vi "appendCsvFile.vi"(8 "error in (no error)":errorcluster, 10 "text to write":string, 11 "Byte Stream File in":refnum<file>) -> (0 "error out":errorcluster)   [LabVIEW 2019]
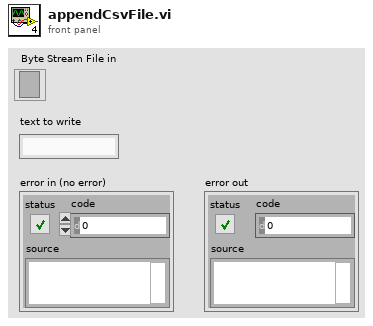
[diagram p1: front panel]
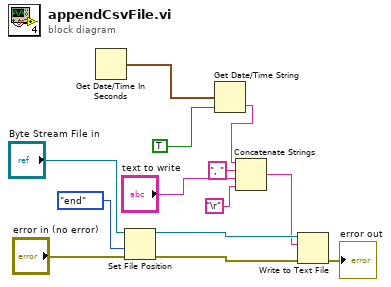
[diagram p0: block diagram]
diagram:
  n1 = Get Date/Time In Seconds() -> (seconds since 1Jan1904=w3:timestamp)
  n2 = Set File Position(refnum="Byte Stream File in", from (0:start)=enum16{"start", "end", "current"}."end", error in="error in (no error)") -> (refnum out=w8:refnum<file>, error out=w10:errorcluster)  [unwired: 1 in]
  n3 = Get Date/Time String(seconds (now)=w3, want seconds? (F)=TRUE) -> (time string=w2:string)  [unwired: 1 in, 1 out]
  n4 = Concatenate Strings(w2, ", " ("string"), "text to write", "\r") -> (w5:string)
  n5 = Write to Text File(file (use dialog)=w8, text=w5, error in=w10) -> (error out=→"error out":errorcluster)  [unwired: 1 in, 2 out]
